vi "onNext.vi"(8 "error in (no error)":errorcluster, 11 "PlayingState in":refnum<class "PlayingState.lvclass">) -> (0 "error out":errorcluster, 2 "String":string, 3 "PlayingState out":refnum<class "PlayingState.lvclass">)   [LabVIEW 2017, in "PlayingState.lvclass"]
uses:
  PlayingState.lvclass
  State Class/State.lvclass
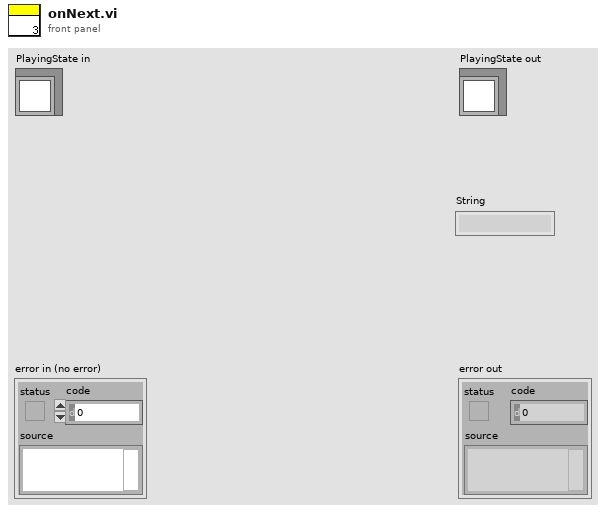
[diagram p1: front panel]
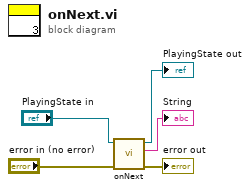
[diagram p0: block diagram]
diagram:
  n1 = call-parent "onNext.vi"("error in (no error)"="error in (no error)", "State in"="PlayingState in") -> ("error out"=→"error out":errorcluster, "String"=→"String":string, "State out"=→"PlayingState out":refnum<class "PlayingState.lvclass">)  [unwired: 7 in]
